vi "BDD_2.vi"(8 "errin":errorcluster, 11 "Cluster":T1={"PN"="00084481", "Sealing"="NANA", "Opérateur"="200", "Conti"="35.000", "OCV"="337", "ISOP"="666.000", "ISOM"="777.000", "1_TCellmin"="1", "1_TCellmax"="2", "1_VCellmin"="3", "1_VCellmax"="4", "1_Nbmodule"="5", "2_TCellmin"="6", "2_TCellmax"="7", "2_VCellmin"="8", "2_VCellmax"="9", "2_Nbmodule"="10", "Résultat final"="1"}) -> (0 "error out":errorcluster, 3 "Chaîne":string)   [LabVIEW 2020]
uses:
  <vilib>/addons/database/Connection.llb/DB Tools Open Connec (String).vi
  <vilib>/addons/database/Connection.llb/Conn Execute.vi
  <vilib>/addons/database/Recordset.llb/Rec Destroy - Connection.vi
  <vilib>/addons/database/NI_Database_API.lvlib
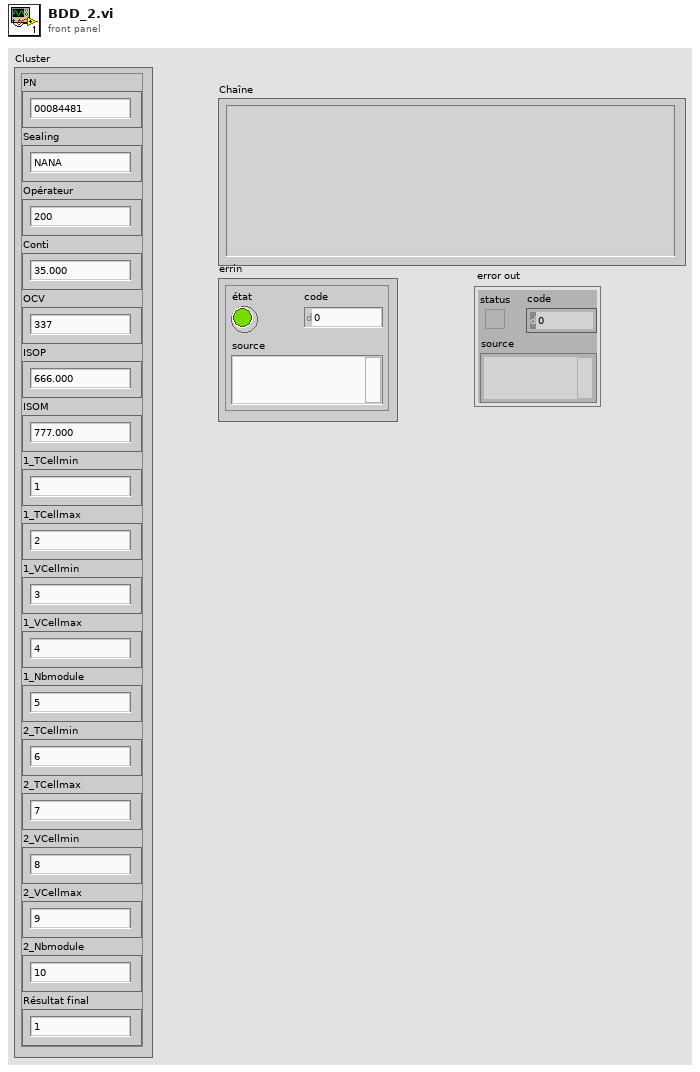
[diagram p1: front panel]
types:
  T1 = cluster{"PN":string, "Sealing":string, "Opérateur":string, "Conti":string, "OCV":string, "ISOP":string, "ISOM":string, "1_TCellmin":string, "1_TCellmax":string, "1_VCellmin":string, "1_VCellmax":string, "1_Nbmodule":string, "2_TCellmin":string, "2_TCellmax":string, "2_VCellmin":string, "2_VCellmax":string, "2_Nbmodule":string, "Résultat final":string}
  T2 = typedef "NI_Database_API.lvlib/Conn ObjectReference.ctl" = refnum<k1>
  T3 = typedef "NI_Database_API.lvlib/Rec ObjectReference.ctl" = refnum<k1>
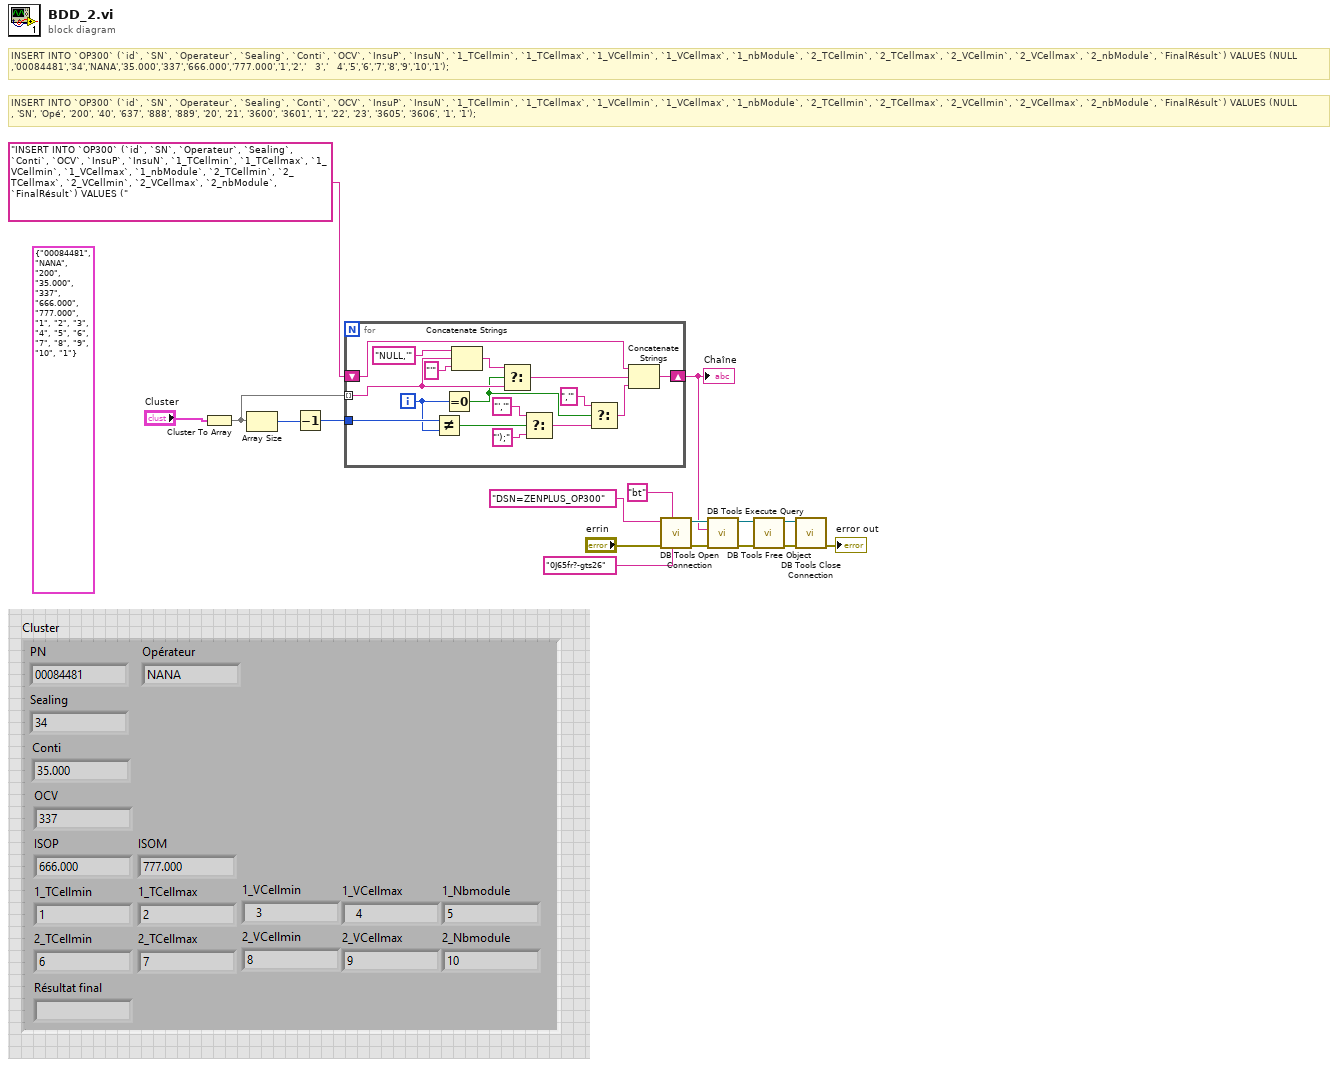
[diagram p0: block diagram]
diagram:
  (unwired) T1 {"PN"="00084481", "Sealing"="NANA", "Opérateur"="200", "Conti"="35.000", "OCV"="337", "ISOP"="666.000", "ISOM"="777.000", "1_TCellmin"="1", "1_TCellmax"="2", "1_VCellmin"="3", "1_VCellmax"="4", "1_Nbmodule"="5", "2_TCellmin"="6", "2_TCellmax"="7", "2_VCellmin"="8", "2_VCellmax"="9", "2_Nbmodule"="10", "Résultat final"="1"} ("Cluster")
  # "INSERT INTO `OP300` (`id`, `SN`, `Operateur`, `Sealing`, `Conti`, `OCV`, `InsuP`, `InsuN`, `1_TCellmin`, `1_TCellmax`, `1_VCellmin`, `1_VCellmax`, `1_nbModule`, `2_TCellmin`, `2_TCellmax`, `2_VCellmin`, `2_VCellmax`, `2_nbModule`, `FinalRésult`) VALUES (NULL\n,'00084481','34','NANA','35.000','337','666.000','777.000','1','2','   3','   4','5','6','7','8','9','10','1');"
  # "INSERT INTO `OP300` (`id`, `SN`, `Operateur`, `Sealing`, `Conti`, `OCV`, `InsuP`, `InsuN`, `1_TCellmin`, `1_TCellmax`, `1_VCellmin`, `1_VCellmax`, `1_nbModule`, `2_TCellmin`, `2_TCellmax`, `2_VCellmin`, `2_VCellmax`, `2_nbModule`, `FinalRésult`) VALUES (NULL\n, 'SN', 'Opé', '200', '40', '637', '888', '889', '20', '21', '3600', '3601', '1', '22', '23', '3605', '3606', '1', '1');"
  n1 = Cluster To Array ("Cluster en tableau")(cluster="Cluster") -> (array=w4:string[])
  n2 = Array Size(array=w4) -> (size(s)=w17:i32)
  n3 = Decrement(x=w17) -> (x-1=w16:i32)
  n4 = for {
    tunnel: w4 -> [w21] mode=indexing
    tunnel: w16 -> [w33]
    shift-right: [w29] -> w6
    shift-left: "INSERT INTO `OP300` (`id`, `SN`, `Operateur`, `Sealing`, `Conti`, `OCV`, `InsuP`, `InsuN`, `1_TCellmin`, `1_TCellmax`, `1_VCellmin`, `1_VCellmax`, `1_nbModule`, `2_TCellmin`, `2_TCellmax`, `2_VCellmin`, `2_VCellmax`, `2_nbModule`, `FinalRésult`) VALUES (" -> [w30]
    i -> [w27]
    n5 = Not Equal?(x=w33, y=w27) -> (x != y?=w32:bool)
    n6 = Equal To 0?(x=w27) -> (x = 0?=w19:bool)
    n7 = Concatenate Strings("NULL,'" ("cas vrai"), w21, "'" ("chaîne")) -> (w20:string)
    n8 = Select(t=w20, s=w19, f=w21) -> (s? t:f=w23:string)
    n9 = Select(t="','" ("chaîne"), s=w32, f="');" ("cas faux")) -> (s? t:f=w28:string)
    n10 = Select(t=",'" ("cas vrai"), s=w19, f=w28) -> (s? t:f=w25:string)
    n11 = Concatenate Strings(w30, w23, w25) -> (w29:string)
  }
  "Chaîne" <- w6
  n12 = call-poly <vilib>:"DB Tools Open Connection.vi"("password"="0J65fr?-gts26", "userID"="bt", "error in (no error)"="errin", "connection information"="DSN=ZENPLUS_OP300") -> ("error out"=w14:errorcluster, "connection reference"=w13:T2)  [unwired: 4 in]
  n13 = call-poly <vilib>:"DB Tools Execute Query.vi"("error in (no error)"=w14, "SQL query"=w6, "connection reference"=w13) -> ("error out"=w10:errorcluster, "recordset reference"=w9:T3)  [unwired: 5 in]
  n14 = call-poly <vilib>:"DB Tools Free Object.vi"("error in (no error)"=w10, "recordset reference"=w9) -> ("error out"=w11:errorcluster, "connection reference"=w12:T2)  [unwired: 8 in]
  n15 = call <vilib>:"DB Tools Close Connection.vi"("error in (no error)"=w11, "connection reference"=w12) -> ("error out"=→"error out":errorcluster)  [unwired: 5 in]
